vi "TRAJECTORY_EXECUTE_SWERVE_OLD.vi"(4 "Time Offset":dbl=-1.0 format="%16.4f", 6 "EnableClosedLoop":bool=TRUE, 7 "Orientation Dmd In":dbl, 8 "Init":bool, 9 "Reverse":bool, 10 "Follow Orientation":bool, 11 "Gyro Heading":dbl) -> (0 "AtReference":bool, 1 "OutputTRAJ_STATE":T6={"TimeSeconds"=0.0, "Velocity"=0.0, "Acceleration"=0.0, "POSE"={"TRANSLATION"={"X"=0.0, "Y"=0.0}, "ROTATION"={"VALUE"=0.0, "COS"=1.0, "SIN"=0.0}}, "Curvature"=0.0} {"POSE"."ROTATION"."SIN" format="%13.4f"; "POSE"."ROTATION"."COS" format="%13.4f"; "POSE"."ROTATION"."VALUE" format="%13.4f"; "POSE"."TRANSLATION"."Y" format="%14.3f"; "POSE"."TRANSLATION"."X" format="%14.3f"}, 2 "Error and Corr":T4 {"Error Pose"."ROTATION"."SIN" format="%13.4f"; "Error Pose"."ROTATION"."COS" format="%13.4f"; "Error Pose"."ROTATION"."VALUE" format="%13.4f"; "Error Pose"."TRANSLATION"."Y" format="%14.3f"; "Error Pose"."TRANSLATION"."X" format="%14.3f"}, 3 "Chassis Velocity Target":T5 {"vOmega" format="%10.3f"; "vY" format="%10.3f"; "vX" format="%10.3f"}, 5 "Orientation Target":dbl)   [LabVIEW 2019]
uses:
  <vilib>/Rock Robotics/WPI/ThirdParty/JAS_Junk/TrajLib/TRAJ_STATE.ctl
  <vilib>/Rock Robotics/WPI/ThirdParty/JAS_Junk/TrajLib/POSE2D.ctl
  <vilib>/Rock Robotics/WPI/ThirdParty/JAS_Junk/TrajLib/TRANSLATION2D.ctl
  <vilib>/Rock Robotics/WPI/ThirdParty/JAS_Junk/TrajLib/ROTATION2D.ctl
  <vilib>/Rock Robotics/WPI/ThirdParty/JAS_Junk/TrajLib/CHASSIS_SPEEDS.ctl
  <vilib>/Rock Robotics/WPI/ThirdParty/JAS_Junk/TrajLib/Translation_Create.vi
  <vilib>/Rock Robotics/WPI/ThirdParty/JAS_Junk/TrajLib/Rotation_UnaryMinus.vi
  <vilib>/Rock Robotics/WPI/ThirdParty/JAS_Junk/TrajLib/Rotation_RotateBy.vi
  <vilib>/Rock Robotics/WPI/ThirdParty/JAS_Junk/TrajLib/PIDController_Calculate_SP_PV.vi
  <vilib>/Rock Robotics/WPI/ThirdParty/JAS_Junk/TrajLib/PIDController_AtSetpoint.vi
  <vilib>/Rock Robotics/WPI/ThirdParty/JAS_Junk/TrajLib/PIDController_SetPID.vi
  <vilib>/Rock Robotics/WPI/ThirdParty/JAS_Junk/TrajLib/PIDController_SetIntegratorRange.vi
  <vilib>/Rock Robotics/WPI/ThirdParty/JAS_Junk/TrajLib/PIDController_SetTolerancePandV.vi
  <vilib>/Rock Robotics/WPI/ThirdParty/JAS_Junk/TrajLib/PIDController_DisableContinousInput.vi
  <vilib>/Rock Robotics/WPI/ThirdParty/JAS_Junk/TrajLib/PIDController_EnableContinousInput.vi
  <vilib>/Rock Robotics/WPI/ThirdParty/JAS_Junk/TrajLib/PIDController_Reset.vi
  <vilib>/Rock Robotics/WPI/ThirdParty/JAS_Junk/TrajLib/PIDController_NewPeriod.vi
  <vilib>/Rock Robotics/WPI/ThirdParty/JAS_Junk/TrajLib/Rotation_GetCos.vi
  <vilib>/Rock Robotics/WPI/ThirdParty/JAS_Junk/TrajLib/Rotation_GetSin.vi
  <vilib>/Rock Robotics/WPI/ThirdParty/JAS_Junk/TrajLib/Rotation_CreateXY.vi
  <vilib>/Rock Robotics/WPI/ThirdParty/JAS_Junk/TrajLib/PIDController_SetSetpoint.vi
  <vilib>/Rock Robotics/WPI/ThirdParty/JAS_Junk/TrajLib/PIDController_Calculate_PV.vi
  <vilib>/Rock Robotics/WPI/ThirdParty/JAS_Junk/TrajLib/ControllerUtil_GetModulusError.vi
  <vilib>/Rock Robotics/SystemInterfaces/NetworkCommunication/NetComm_UsageReport_report.vi
  <vilib>/Rock Robotics/WPI/ThirdParty/JAS_Junk/TrajLib/Util_CalcDist.vi
  <vilib>/Rock Robotics/WPI/ThirdParty/JAS_Junk/TrajLib/Util_LibraryGlobals.vi
  <vilib>/Rock Robotics/WPI/ThirdParty/JAS_Junk/TrajLib/Trajectory_Library.lvlib
panel:
  # "(FOR TESTING)"
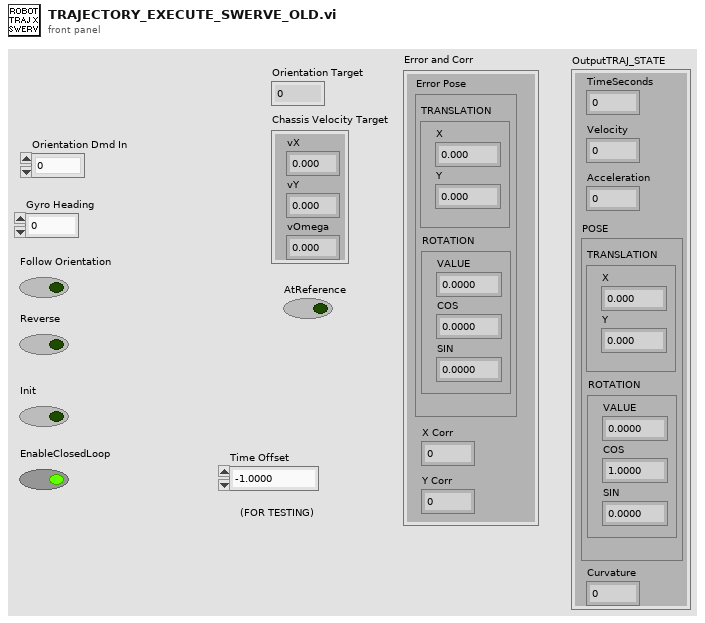
[diagram p1: front panel]
types:
  T1 = typedef "Trajectory_Library.lvlib/POSE2D.ctl" = cluster{"TRANSLATION":T2, "ROTATION":T3}
  T2 = typedef "Trajectory_Library.lvlib/TRANSLATION2D.ctl" = cluster{"X":dbl, "Y":dbl}
  T3 = typedef "Trajectory_Library.lvlib/ROTATION2D.ctl" = cluster{"VALUE":dbl, "COS":dbl, "SIN":dbl}
  T4 = cluster{"Error Pose":T1, "X Corr":dbl, "Y Corr":dbl}
  T5 = typedef "Trajectory_Library.lvlib/CHASSIS_SPEEDS.ctl" = cluster{"vX":dbl, "vY":dbl, "vOmega":dbl}
  T6 = typedef "Trajectory_Library.lvlib/TRAJ_STATE.ctl" = cluster{"TimeSeconds":dbl, "Velocity":dbl, "Acceleration":dbl, "POSE":T1, "Curvature":dbl}
  T7 = typedef "Trajectory_Library.lvlib/SWERVE_DRIVE_KINEMATICS.ctl" = cluster{"NumModules":i32, "InverseKinematics":T8, "ForwardKinematics":T8, "Modules":T2[], "PrevCoR":T2}
  T8 = typedef "NI_Matrix.lvlib/RealMatrix.ctl" = dbl[][]
  T9 = typedef "Trajectory_Library.lvlib/SWERVE_DRIVE_ODOMETRY.ctl" = cluster{"POSE":T1, "GyroOffset":T3, "PreviousAngle":T3, "PrevTime":dbl}
  T10 = typedef "Trajectory_Library.lvlib/TRAJECTORY.ctl" = cluster{"TotalTImeSecs":dbl, "States":T6[]}
  T11 = typedef "Trajectory_Library.lvlib/SWERVE_DRIVE_MODULE_STATE.ctl" = cluster{"Speed":dbl, "Angle":T3}
  T12 = typedef "Trajectory_Library.lvlib/PID_TUNING.ctl" = cluster{"Kp":dbl, "Ki":dbl, "Kd":dbl, "MaximumIntegral":dbl, "MinimumIntegral":dbl}
  T13 = typedef "Trajectory_Library.lvlib/PID_ERROR_TOLERANCE.ctl" = cluster{"PositionTolerance":dbl, "VelocityTolerance":dbl}
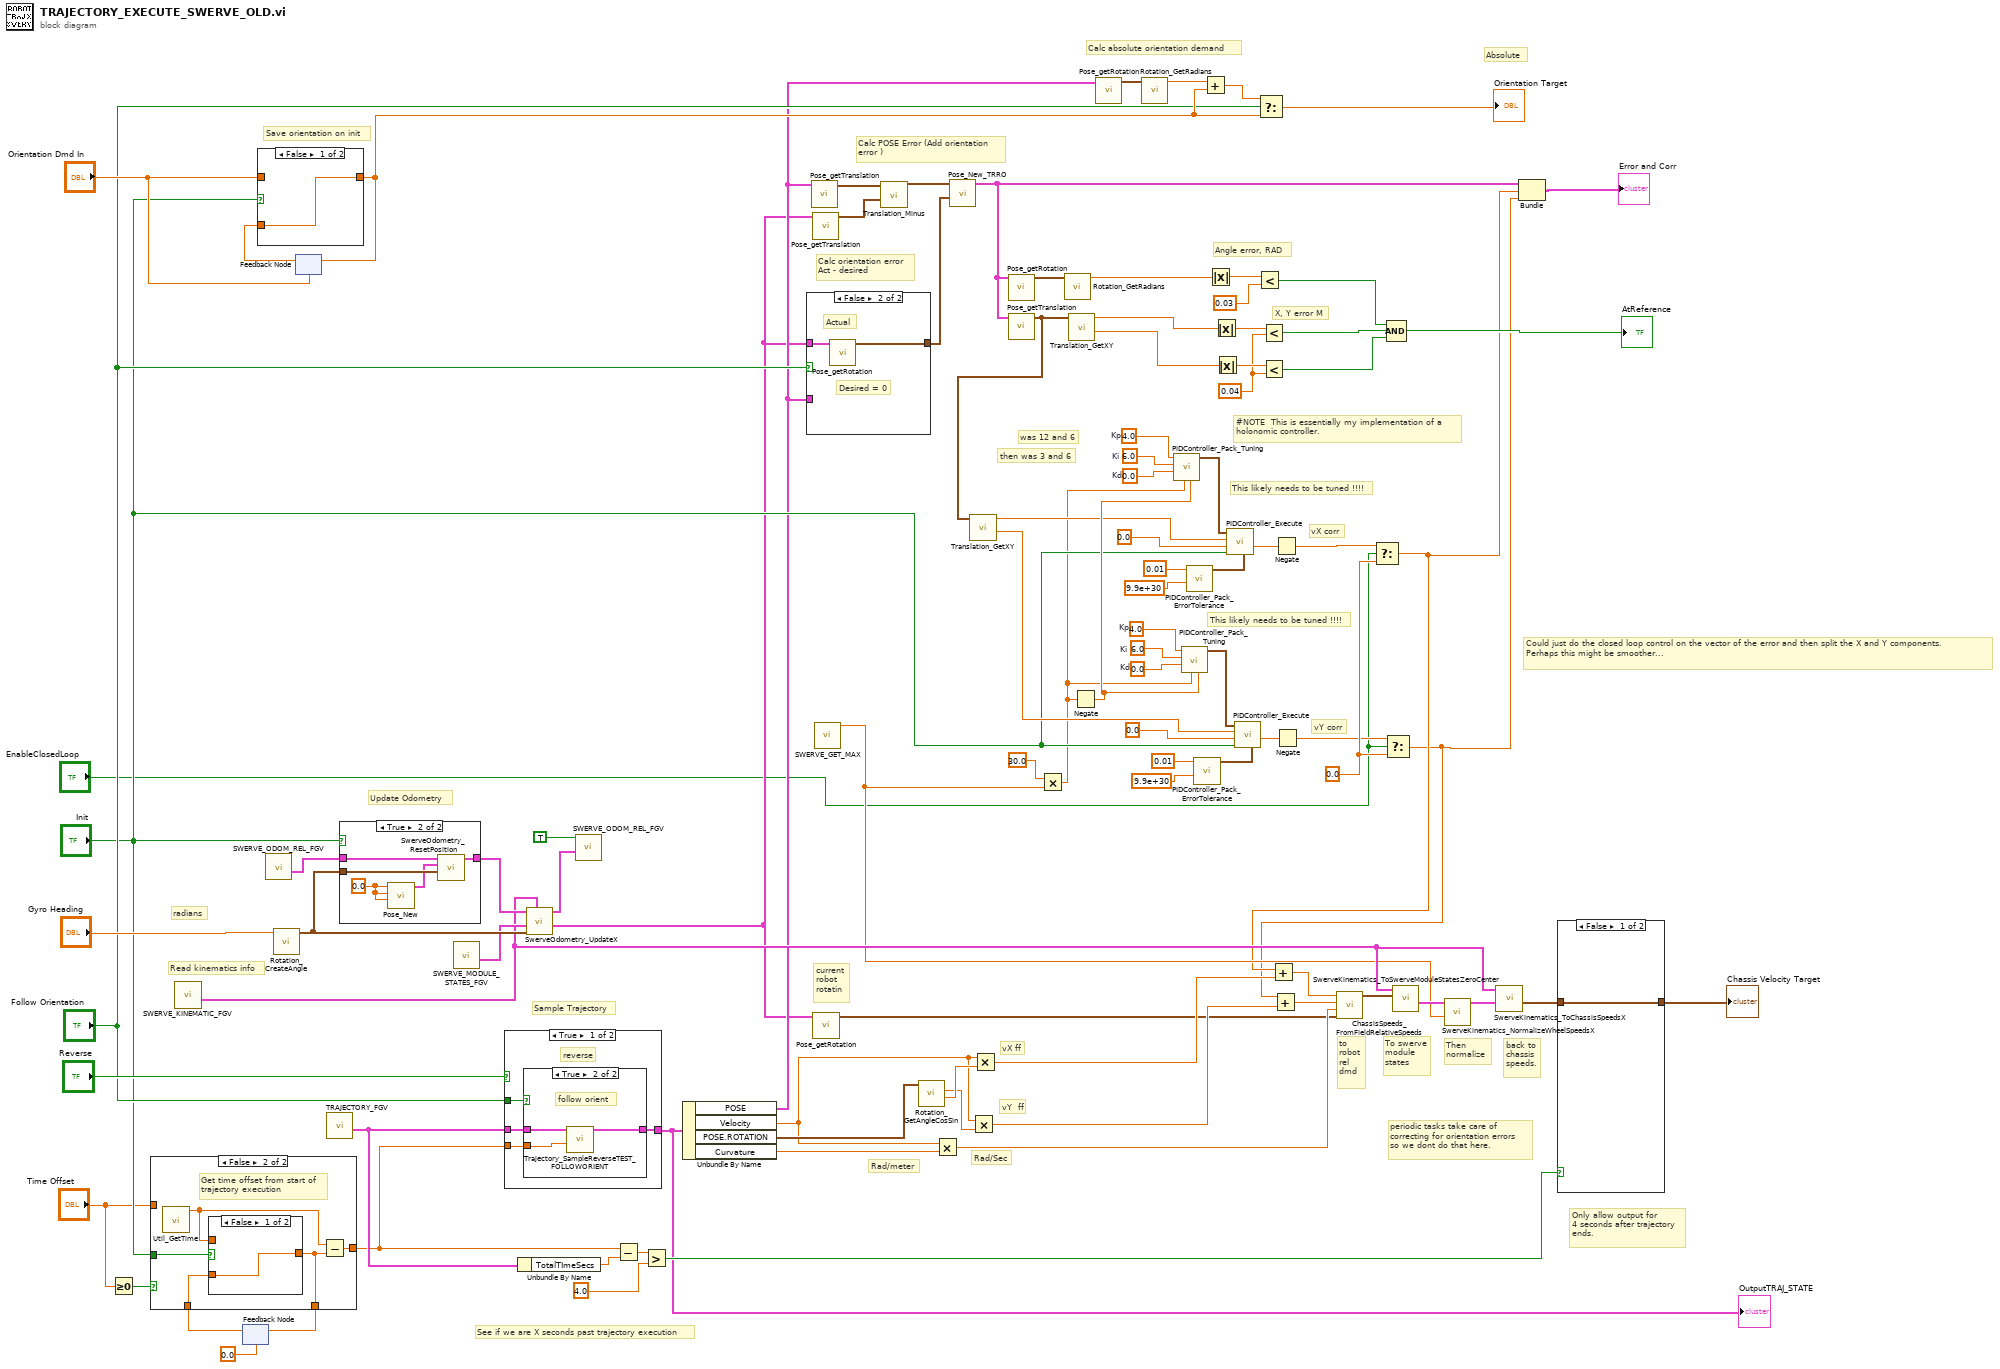
[diagram p0: block diagram]
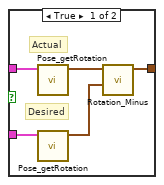
[diagram p4: hidden frame]
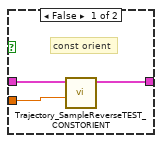
[diagram p5: hidden frame]
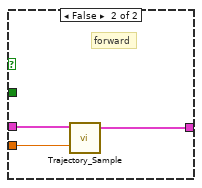
[diagram p6: hidden frame]
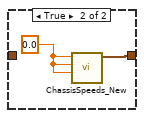
[diagram p9: hidden frame]
diagram:
  w40 = 0.0  # Kd
  w41 = 6.0  # Ki
  w42 = 4.0  # Kp
  w49 = 0.0  # Kd
  w50 = 6.0  # Ki
  w51 = 4.0  # Kp
  w59 = 0.0 ("f")
  w81 = 0.04
  # "#NOTE  This is essentially my implementation of a\nholonomic controller."
  # "Angle error, RAD"
  # "X, Y error M"
  # "then was 3 and 6"
  # "was 12 and 6"
  # "to\nrobot\nrel\ndmd"
  # "This likely needs to be tuned !!!!"
  # "This likely needs to be tuned !!!!"
  # "Could just do the closed loop control on the vector of the error and then split the X and Y components.  \nPerhaps this might be smoother..."
  # "vY corr"
  # "vX corr"
  # "current\nrobot\nrotatin"
  # "vY  ff"
  # "vX ff"
  # "back to\nchassis\nspeeds."
  # "Then\nnormalize"
  # "To swerve\nmodule\nstates"
  # "Rad/Sec"
  # "Rad/meter"
  # "Calc POSE Error (Add orientation\nerror )"
  # "Calc orientation error\nAct - desired"
  # "Calc absolute orientation demand"
  # "Read kinematics info"
  # "Sample Trajectory"
  # "See if we are X seconds past trajectory execution"
  # "Save orientation on init"
  # "Absolute"
  # "Update Odometry"
  # "radians"
  # "periodic tasks take care of\ncorrecting for orientation errors\nso we dont do that here."
  # "Only allow output for\n4 seconds after trajectory\nends."
  n1 = Greater Or Equal To 0?(x="Time Offset") -> (x >= 0?=w6:bool)
  n2 = call "SWERVE_KINEMATIC_FGV.vi"() -> ("out SWERVE_DRIVE_KINEMATICS"=w74:T7)  [unwired: 11 in]
  n3 = feedback #1(0.0 ("TIME")) -> (w8:dbl)
  n4 = case shown="False" w6 {
    tunnel: [w99 w105] -> w96
    tunnel: "Init" -> [_ w103]
    tunnel: w8 -> [w100 w102]
    tunnel: [w100 w101] -> w7
    tunnel: "Time Offset" -> [w99 _]
    frame True {
      # "For testing allow\nuser entered time offset!!"
    }
    frame False {
      # "Get time offset from start of\ntrajectory execution"
      n5 = call <vilib>:"Util_GetTime.vi"() -> ("FPGA_Time_Seconds"=w104:dbl)  [unwired: 10 in, 1 out]
      n6 = case shown="False" w103 {
        tunnel: [w106 w107] -> w101
        tunnel: w102 -> [w106 _]
        tunnel: w104 -> [_ w107]
        frame False {
        }
        frame True {
        }
      }
      n7 = Subtract(x=w104, y=w101) -> (x-y=w105:dbl)
    }
  }
  n8 = feedback-in #1(w7) -> ()
  n9 = call "SWERVE_ODOM_REL_FGV.vi"() -> ("out SWERVE_DRIVE_ODOMETRY"=w91:T9)  [unwired: 11 in]
  n10 = call <vilib>:"Rotation_CreateAngle.vi"("Angle"="Gyro Heading") -> ("ROTATION"=w89:T3)  [unwired: 10 in]
  n11 = feedback #2("Orientation Dmd In") -> (w72:dbl)
  n12 = case shown="False" "Init" {
    tunnel: "Orientation Dmd In" -> [_ w109]
    tunnel: [w108 w109] -> w69
    tunnel: w72 -> [w108 _]
    frame False {
    }
    frame True {
    }
  }
  n13 = feedback-in #2(w69) -> ()
  n14 = call "TRAJECTORY_FGV.vi"() -> ("outTRAJECTORY"=w98:T10)  [unwired: 11 in]
  n15 = case shown="True" "Init" {
    tunnel: w91 -> [w110 w115]
    tunnel: [w110 w114] -> w90
    tunnel: w89 -> [_ w113]
    frame False {
    }
    frame True {
      w112 = 0.0 ("X")
      n16 = call <vilib>:"Pose_New.vi"("Heading"=w112, "Y"=w112, "X"=w112) -> ("out POSe"=w111:T1)  [unwired: 8 in]
      n17 = call <vilib>:"SwerveOdometry_ResetPosition.vi"("gyroAngle"=w113, "Pose"=w111, "in SWERVE_DRIVE_ODOMETRY"=w115) -> ("out SWERVE_DRIVE_ODOMETRY"=w114:T9)  [unwired: 8 in]
    }
  }
  n18 = call "SWERVE_MODULE_STATES_FGV.vi"() -> ("out Current Module States"=w87:T11[])  [unwired: 11 in]
  n19 = case shown="True" "Reverse" {
    tunnel: w98 -> [w119 w128]
    tunnel: w96 -> [w117 w127]
    tunnel: [w118 w126] -> w86
    tunnel: "Follow Orientation" -> [w116 _]
    frame True {
      # "reverse"
      n20 = case shown="True" w116 {
        tunnel: w119 -> [w122 w125]
        tunnel: [w120 w124] -> w118
        tunnel: w117 -> [w121 w123]
        frame False {
          # "const orient"
          n21 = call "Trajectory_SampleReverseTEST_CONSTORIENT.vi"("Time"=w121, "InputTRAJECTORY"=w122) -> ("OutputTRAJ_STATE"=w120:T6)  [unwired: 9 in]
        }
        frame True {
          # "follow orient"
          n22 = call "Trajectory_SampleReverseTEST_FOLLOWORIENT.vi"("Time"=w123, "InputTRAJECTORY"=w125) -> ("OutputTRAJ_STATE"=w124:T6)  [unwired: 9 in]
        }
      }
    }
    frame False {
      # "forward"
      n23 = call <vilib>:"Trajectory_Sample.vi"("Time"=w127, "InputTRAJECTORY"=w128) -> ("OutputTRAJ_STATE"=w126:T6)  [unwired: 9 in]
    }
  }
  "OutputTRAJ_STATE" <- w86
  n24 = Unbundle By Name(w98) -> ("TotalTImeSecs"=w97:dbl)
  n25 = call <vilib>:"SwerveOdometry_UpdateX.vi"("SWERVE_DRIVE_KINEMATICS"=w74, "gyroAngle"=w89, "module States"=w87, "in SWERVE_DRIVE_ODOMETRY"=w90) -> ("robot POSE"=w14:T1, "out SWERVE_DRIVE_ODOMETRY"=w65:T9)  [unwired: 6 in]
  n26 = call "SWERVE_ODOM_REL_FGV.vi"("in SWERVE_DRIVE_ODOMETRY"=w65, "WRITE"=TRUE) -> ()  [unwired: 9 in, 1 out]
  n27 = Subtract(x=w96, y=w97) -> (x-y=w95:dbl)
  n28 = Greater?(x=w95, y=4.0) -> (0:w93:bool)
  n29 = Unbundle By Name(w86) -> ("POSE"=w15:T1, "Velocity"=w24:dbl, "POSE.ROTATION"=w27:T3, "Curvature"=w64:dbl)
  n30 = case shown="False" "Follow Orientation" {
    tunnel: w14 -> [w133 w135]
    tunnel: w15 -> [w132 _]
    tunnel: [w129 w134] -> w60
    frame True {
      # "Desired"
      # "Actual"
      n31 = call <vilib>:"Pose_getRotation.vi"("in POSE"=w133) -> ("out ROTATION"=w131:T3)  [unwired: 10 in]
      n32 = call <vilib>:"Pose_getRotation.vi"("in POSE"=w132) -> ("out ROTATION"=w130:T3)  [unwired: 10 in]
      n33 = call <vilib>:"Rotation_Minus.vi"("other ROTATION"=w130, "in ROTATION"=w131) -> ("out ROTATION"=w129:T3)  [unwired: 9 in]
    }
    frame False {
      # "Desired = 0"
      # "Actual"
      n34 = call <vilib>:"Pose_getRotation.vi"("in POSE"=w135) -> ("out ROTATION"=w134:T3)  [unwired: 10 in]
    }
  }
  n35 = call <vilib>:"Pose_getTranslation.vi"("in POSE"=w15) -> ("outTRANSLATION"=w13:T2)  [unwired: 10 in]
  n36 = call <vilib>:"Pose_getTranslation.vi"("in POSE"=w14) -> ("outTRANSLATION"=w12:T2)  [unwired: 10 in]
  n37 = call <vilib>:"Pose_getRotation.vi"("in POSE"=w14) -> ("out ROTATION"=w17:T3)  [unwired: 10 in]
  n38 = call "SWERVE_GET_MAX.vi"() -> ("Max Wheel Vel (Meter/Sec)"=w37:dbl)  [unwired: 10 in, 1 out]
  n39 = call <vilib>:"Translation_Minus.vi"("other Translation"=w12, "In Translation"=w13) -> ("Out Translation"=w11:T2)  [unwired: 9 in]
  n40 = call <vilib>:"Rotation_GetAngleCosSin.vi"("in ROTATION"=w27) -> ("Cosine"=w26:dbl, "Sine"=w25:dbl)  [unwired: 8 in, 1 out]
  n41 = Multiply(x=w24, y=w64) -> (x*y=w18:dbl)
  n42 = call <vilib>:"Pose_New_TRRO.vi"("ROTATION"=w60, "TRANSLATION"=w11) -> ("outPOSE"=w4:T1)  [unwired: 9 in]
  n43 = Multiply(x=w24, y=w25) -> (x*y=w23:dbl)
  n44 = Multiply(x=w24, y=w26) -> (x*y=w22:dbl)
  n45 = call <vilib>:"Pose_getRotation.vi"("in POSE"=w4) -> ("out ROTATION"=w55:T3)  [unwired: 10 in]
  n46 = call <vilib>:"Pose_getTranslation.vi"("in POSE"=w4) -> ("outTRANSLATION"=w21:T2)  [unwired: 10 in]
  n47 = call <vilib>:"Translation_GetXY.vi"("In Translation"=w21) -> ("Y"=w34:dbl, "X"=w35:dbl)  [unwired: 9 in]
  n48 = Multiply(x=30.0, y=w37) -> (x*y=w28:dbl)
  n49 = call <vilib>:"Rotation_GetRadians.vi"("in ROTATION"=w55) -> ("AngleRadians"=w57:dbl)  [unwired: 10 in]
  n50 = call <vilib>:"Translation_GetXY.vi"("In Translation"=w21) -> ("Y"=w56:dbl, "X"=w58:dbl)  [unwired: 9 in]
  n51 = Negate(x=w28) -> (-x=w36:dbl)
  n52 = call <vilib>:"Pose_getRotation.vi"("in POSE"=w15) -> ("out ROTATION"=w70:T3)  [unwired: 10 in]
  n53 = call <vilib>:"Rotation_GetRadians.vi"("in ROTATION"=w70) -> ("AngleRadians"=w68:dbl)  [unwired: 10 in]
  n54 = call <vilib>:"PIDController_Pack_Tuning.vi"("MinimumIntegral"=w36, "MaximumIntegral"=w28, "Kd"=w49, "Ki"=w50, "Kp"=w51) -> ("PID Tuning"=w54:T12)  [unwired: 6 in]
  n55 = call <vilib>:"PIDController_Pack_Tuning.vi"("MinimumIntegral"=w36, "MaximumIntegral"=w28, "Kd"=w40, "Ki"=w41, "Kp"=w42) -> ("PID Tuning"=w45:T12)  [unwired: 6 in]
  n56 = call <vilib>:"PIDController_Pack_ErrorTolerance.vi"("VelocityTolerance"=9.9e+30, "PositionTolerance"=0.01) -> ("PID Error Tolerance"=w52:T13)  [unwired: 9 in]
  n57 = call <vilib>:"PIDController_Pack_ErrorTolerance.vi"("VelocityTolerance"=9.9e+30, "PositionTolerance"=0.01) -> ("PID Error Tolerance"=w43:T13)  [unwired: 9 in]
  n58 = Add(x=w68, y=w69) -> (x+y=w67:dbl)
  n59 = Absolute Value(x=w57) -> (abs(x)=w85:dbl)
  n60 = Absolute Value(x=w58) -> (abs(x)=w84:dbl)
  n61 = Absolute Value(x=w56) -> (abs(x)=w83:dbl)
  n62 = call <vilib>:"PIDController_Execute.vi"("PID Error Tolerance"=w52, "Reset"="Init", "SP-SetPoint"=0.0, "PV-Measurement"=w35, "PID Tuning"=w54) -> ("CO-ControlOutput"=w33:dbl)  [unwired: 4 in, 2 out]
  n63 = call <vilib>:"PIDController_Execute.vi"("PID Error Tolerance"=w43, "Reset"="Init", "SP-SetPoint"=0.0, "PV-Measurement"=w34, "PID Tuning"=w45) -> ("CO-ControlOutput"=w32:dbl)  [unwired: 4 in, 2 out]
  n64 = Less?(x=w85, y=0.03) -> (x < y?=w80:bool)
  n65 = Select(t=w67, s="Follow Orientation", f=w69) -> (s? t:f=→"Orientation Target":dbl)
  n66 = Less?(x=w84, y=w81) -> (x < y?=w79:bool)
  n67 = Less?(x=w83, y=w81) -> (x < y?=w78:bool)
  n68 = Negate(x=w33) -> (-x=w31:dbl)
  n69 = Negate(x=w32) -> (-x=w30:dbl)
  n70 = Select(t=w31, s="EnableClosedLoop", f=w59) -> (s? t:f=w3:dbl)
  n71 = Add(x=w3, y=w22) -> (x+y=w20:dbl)
  n72 = Select(t=w30, s="EnableClosedLoop", f=w59) -> (s? t:f=w2:dbl)
  n73 = Add(x=w2, y=w23) -> (x+y=w19:dbl)
  n74 = call <vilib>:"ChassisSpeeds_FromFieldRelativeSpeeds.vi"("RobotAngle"=w17, "Omega"=w18, "vY"=w19, "vX"=w20) -> ("CHASSIS"=w16:T5)  [unwired: 7 in]
  n75 = Compound Arithmetic op=AND(w80, w79, w78) -> (→"AtReference":bool)
  n76 = call <vilib>:"SwerveKinematics_ToSwerveModuleStatesZeroCenter.vi"("ChassisSpeeds"=w16, "in SWERVE_DRIVE_KINEMATICS"=w74) -> ("ModuleStates"=w76:T11[])  [unwired: 8 in, 1 out]
  n77 = call <vilib>:"SwerveKinematics_NormalizeWheelSpeedsX.vi"("AttainableMaxSpeed"=w37, "in WheelStates"=w76) -> ("out WheelStates"=w75:T11[])  [unwired: 9 in]
  n78 = call <vilib>:"SwerveKinematics_ToChassisSpeedsX.vi"("WheelStates"=w75, "in SWERVE_DRIVE_KINEMATICS"=w74) -> ("Chassis Speed"=w62:T5)  [unwired: 9 in]
  n79 = Bundle("outPOSE"=w4, "f"=w3, "f"=w2) -> (→"Error and Corr":cluster{"outPOSE":T1, "f":dbl, "f":dbl})  [unwired: 1 in]
  n80 = case shown="False" w93 {
    tunnel: w62 -> [w136 _]
    tunnel: [w136 w137] -> w61
    frame False {
    }
    frame True {
      w138 = 0.0 ("vX")
      n81 = call <vilib>:"ChassisSpeeds_New.vi"("vAngular"=w138, "vY"=w138, "vX"=w138) -> ("CHASSIS"=w137:T5)  [unwired: 8 in]
    }
  }
  "Chassis Velocity Target" <- w61
